vi "SetMotors.vi"(0 "Position Motors":T4[](array[typedef]), 1 "Speed Motors":T4[](array[typedef]), 3 "Angle (radians; 0 = right)":dbl, 4 "Trigger Axes":cluster{"Left":dbl, "Right":dbl}, 5 "Strafe Joystick Axes":cluster{"X":dbl, "Y":dbl}, 6 "error in (no error)":errorcluster, 7 "Face Joystick Axes":cluster{"X":dbl, "Y":dbl}, 8 "Absolute Encoder TPR":dbl, 9 "Rotation Multipliers":T1, 10 "Rotation Angle Cluster":T2 {"FL Angle" scale=3.1416..-3.1416; "FR Angle" scale=3.1416..-3.1416; "RR Angle" scale=3.1416..-3.1416; "RL Angle" scale=3.1416..-3.1416}, 11 "Drive Train Absolute Offsets (ticks)":dbl[](array[numeric])=[-0.395, 1.11, 1.68, -1.896], 12 "Speed Multipliers":dbl=1.0) -> (13 "error out":errorcluster)   [LabVIEW 2015]
uses:
  <vilib>/Rock Robotics/WPI/MotorControl/WPI_MotorControlDeviceRef.ctl
  <vilib>/Rock Robotics/WPI/MotorControl/WPI_MotorControlType.ctl
  <vilib>/Rock Robotics/SystemInterfaces/DIO/FPGA_DIOPWMChannel.ctl
  <vilib>/Rock Robotics/WPI/PWM/WPI_PWMDeadband.ctl
  <vilib>/Rock Robotics/WPI/CAN/Jaguar/SubVIs/WPI_CANJaguar_ControlMode.ctl
  <vilib>/Rock Robotics/WPI/CAN/TalonSRX/WPI_CANTalonSRX_APIControlMode.ctl
  <vilib>/addons/control/pid/pid.llb/PID Control Input Filter (DBL).vi
  <vilib>/addons/control/pid/pid.llb/PID (DBL).vi
  <vilib>/addons/control/pid/NI_PID_pid.lvlib
panel:
  out "Position Output":dbl
  out "Speed Output":dbl
  in  "Max Wheel Speed":dbl=20000.0
  in  "Face PID Gains":T3 {"derivative time (Td, min)" format="%.3f"; "integral time (Ti, min)" format="%.3f"; "proportional gain (Kc)" format="%.3f"}
  out "Speed Chart":cluster{dbl, "Encoder Velocity":dbl}[](graph)
  out "Position Chart":cluster{dbl, "Encoder Velocity":dbl}[](graph)
  out "Speed Cluster":T11 {"RR Speed" scale=-1.0..1.0; "RL Speed" scale=-1.0..1.0; "FR Speed" scale=-1.0..1.0; "FL Speed" scale=-1.0..1.0}
  out "Angle Cluster":T2 {"FL Angle" scale=3.1416..-3.1416; "FR Angle" scale=3.1416..-3.1416; "RR Angle" scale=3.1416..-3.1416; "RL Angle" scale=3.1416..-3.1416}
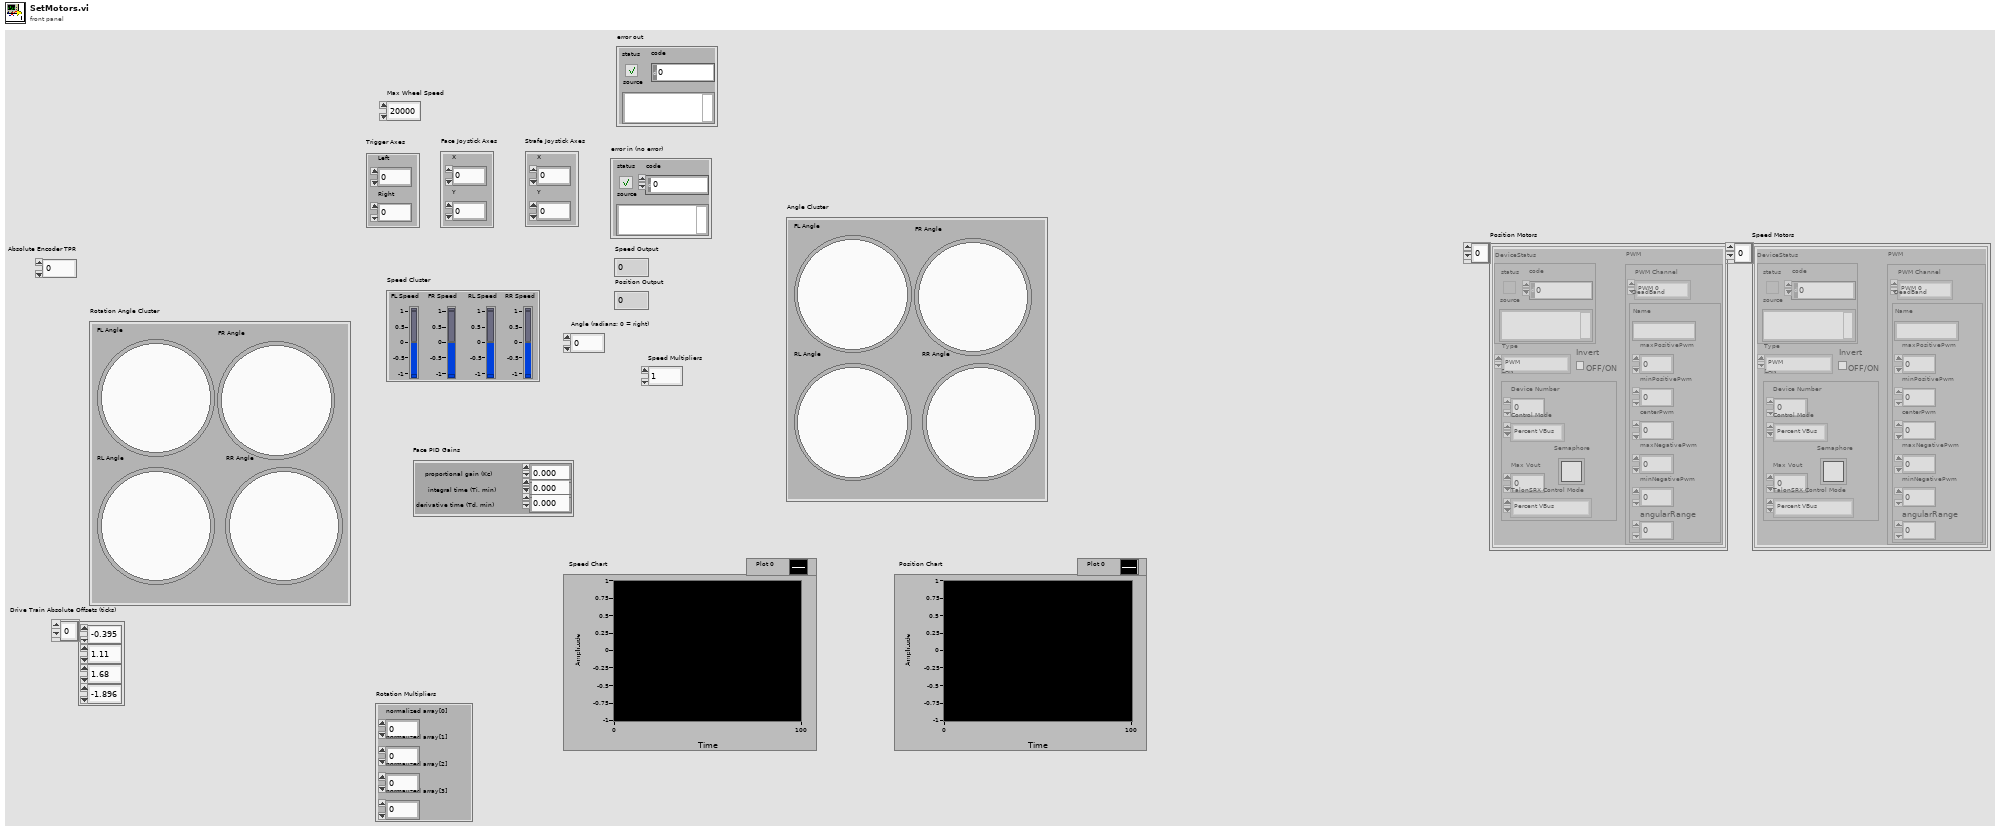
[diagram p1: front panel]
types:
  T1 = cluster{"normalized array[0]":dbl, "normalized array[1]":dbl, "normalized array[2]":dbl, "normalized array[3]":dbl}
  T2 = cluster{"FL Angle":dbl, "FR Angle":dbl, "RL Angle":dbl, "RR Angle":dbl}
  T3 = cluster{"proportional gain (Kc)":dbl, "integral time (Ti, min)":dbl, "derivative time (Td, min)":dbl}
  T4 = typedef "WPI_MotorControlDeviceRef.ctl" = cluster{"DeviceStatus":errorcluster, "Type":T5, "PWM":cluster{"PWM Channel":T6, "DeadBand":T7}, "CAN":cluster{"Device Number":u8, "Control Mode":T8, "Semaphore":T9, "Max Vout":dbl, "TalonSRX Control Mode":T10}, "Invert":bool}
  T5 = typedef "WPI_MotorControlType.ctl" = enum16{"PWM", "CAN", "CANTalonSRX"}
  T6 = typedef "FPGA_DIOPWMChannel.ctl" = enum8{"PWM 0", "PWM 1", "PWM 2", "PWM 3", "PWM 4", "PWM 5", "PWM 6", "PWM 7", "PWM 8", "PWM 9", "PWM MXP 0", "PWM MXP 1", "PWM MXP 2", "PWM MXP 3", "PWM MXP 4", "PWM MXP 5", "PWM MXP 6", "PWM MXP 7", "PWM MXP 8", "PWM MXP 9", "Invalid"}
  T7 = typedef "WPI_PWMDeadband.ctl" = cluster{"Name":string, "maxPositivePwm":i32, "minPositivePwm":i32, "centerPwm":i32, "maxNegativePwm":i32, "minNegativePwm":i32, "angularRange":u16}
  T8 = typedef "WPI_CANJaguar_ControlMode.ctl" = enum8{"Percent VBus", "Current", "Speed", "Position", "Voltage"}
  T9 = typedef "Semaphore RefNum" = refnum<k1>
  T10 = typedef "WPI_CANTalonSRX_APIControlMode.ctl" = enum8{"Percent VBus", "Speed", "Position", "Slave", "Unchanged / Invalid", "Voltage Compensation", "Current"}
  T11 = cluster{"FL Speed":dbl, "FR Speed":dbl, "RL Speed":dbl, "RR Speed":dbl}
  T12 = cluster{"[0]":dbl, "[1]":dbl, "[2]":dbl, "[3]":dbl}
  T13 = typedef "WPI_CANTalonSRX_GlobalStatus.ctl" = cluster{"Applied Throttle":dbl, "Module Enabled":bool, "CAN Error":errorcluster, "Closed Loop Error":dbl, "Forward Limit Switch Closed":bool, "Reverse Limit Switch Closed":bool, "Sensor Position":dbl, "Sensor Velocity":dbl, "Current":dbl, "Sticky Fault - Over Temp":bool, "Sticky Fault - Under Voltage":bool, "Sticky Fault - Forward Limit":bool, "Sticky Fault - Reverse Limit":bool, "Sticky Fault - Forward Soft Limit":bool, "Sticky Fault - Reverse Soft Limit":bool, "Brake is Enabled":bool, "Encoder Position":dbl, "Encoder Velocity":dbl, "Encoder Index Count":dbl, "Encoder A Pin State":bool, "Encoder B Pin State":bool, "Encoder Index Pin State":bool, "Analog In":dbl, "Analog In Velocity":dbl, "Temperature (C)":dbl, "Battery Voltage":dbl}
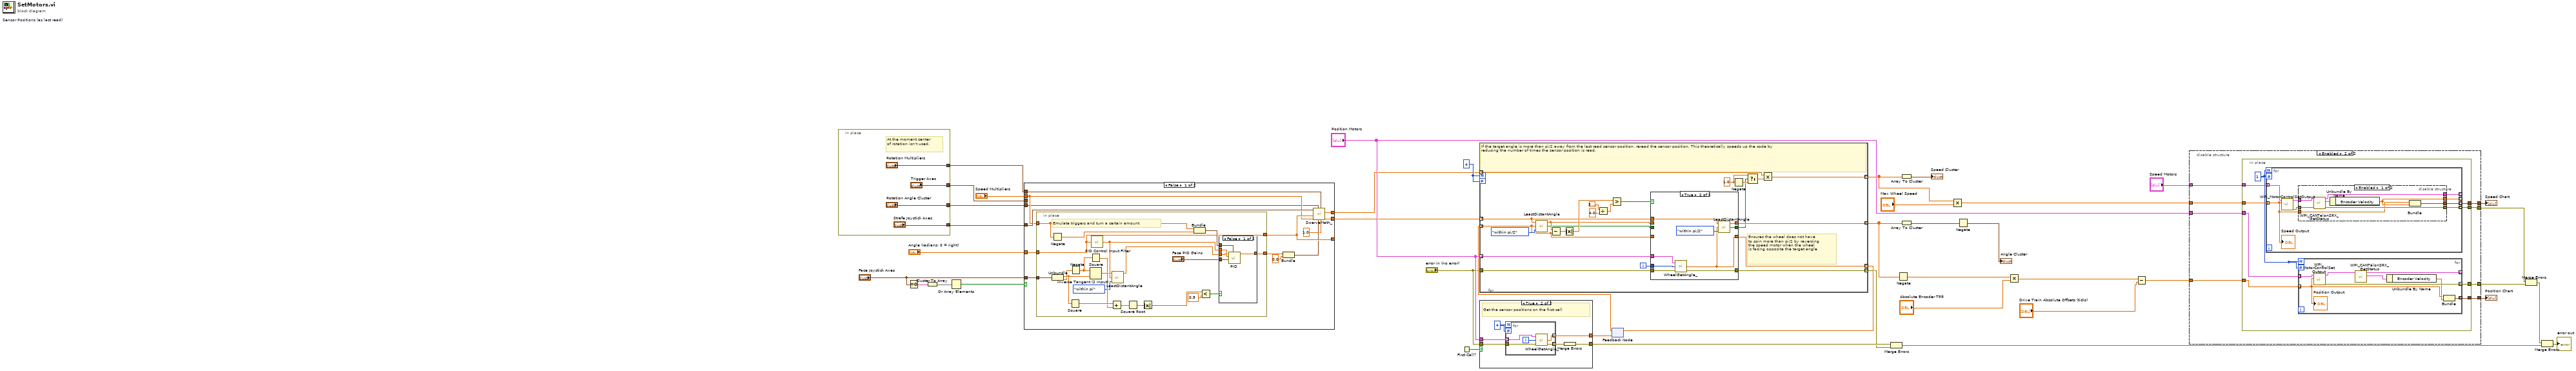
[diagram p0: block diagram]
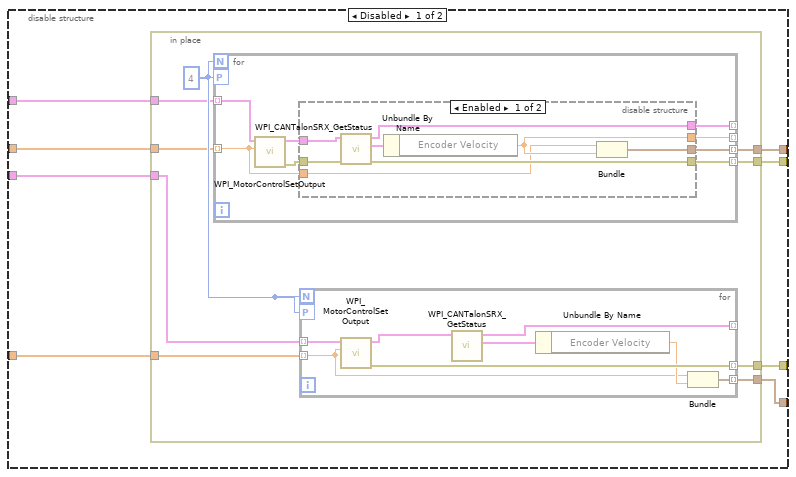
[diagram p2: hidden frame]
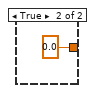
[diagram p7: hidden frame]
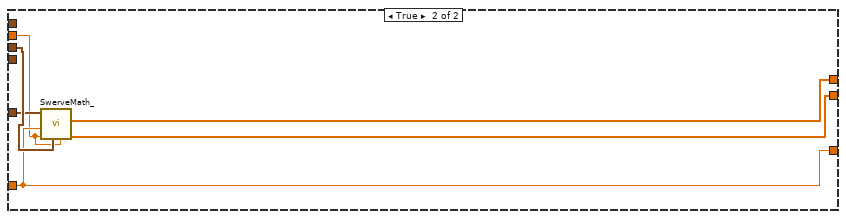
[diagram p8: hidden frame]
diagram:
  w29 = 4
  n1 = in-place {
    in-place-border: ["Strafe Joystick Axes"] -> w13
    in-place-border: ["Trigger Axes"] -> w9
    in-place-border: ["Rotation Multipliers"] -> w4
    in-place-border: ["Rotation Angle Cluster"] -> w3
    # "At the moment center\nof rotation isn't used."
  }
  n2 = Equal To 0?(x="Face Joystick Axes") -> (x = 0?=w32:cluster{"X":bool, "Y":bool})
  n3 = Cluster To Array(cluster=w32) -> (array=w30:bool[])
  n4 = Or Array Elements(Boolean array=w30) -> (logical OR=w31:bool)
  n5 = case shown="False" w31 {
    tunnel: "Face Joystick Axes" -> [w58 _]
    tunnel: [w53 w89] -> _
    tunnel: "Angle (radians; 0 = right)" -> [w57 w89]
    tunnel: w13 -> [w54 w90]
    tunnel: [w51 w88] -> w11
    tunnel: [w50 w87] -> w12
    tunnel: "Speed Multipliers" -> [w48 w86]
    tunnel: w9 -> [_ w91]
    tunnel: w4 -> [w47 _]
    tunnel: w3 -> [w46 _]
    frame False {
      n6 = in-place {
        in-place-border: [w79] -> w56
        in-place-border: [w60] -> w53
        in-place-border: w58 -> [w62]
        in-place-border: w57 -> [w60]
        in-place-border: w48 -> [w59]
        # "Emulate triggers and turn a certain amount"
        n7 = Negate(x=w59) -> (-x=w68:dbl)
        n8 = Unbundle(w62) -> ("X"=w73:dbl, "Y"=w72:dbl)
        n9 = Square(x=w73) -> (x^2=w77:dbl)
        n10 = Negate(x=w72) -> (-x=w69:dbl)
        n11 = Square(x=w69) -> (x^2=w76:dbl)
        n12 = Inverse Tangent (2 Input)(1:w73, 2:w69) -> (0:w65:dbl)
        n13 = call-poly <vilib>:"PID Control Input Filter.vi"("input"=w60) -> ("output"=w63:dbl)  [unwired: 4 in]
        n14 = Add(x=w77, y=w76) -> (x+y=w75:dbl)
        n15 = call "LeastDistantAngle.vi"("Enum"=enum16{"within pi", "within pi/2"}."within pi", "Current angle"=w63, "target angle (between pi and -pi)"=w65) -> ("output angle"=w61:dbl)  [unwired: 2 out]
        n16 = Square Root(x=w75) -> (sqrt(x)=w74:dbl)
        n17 = Absolute Value(x=w74) -> (abs(x)=w70:dbl)
        n18 = Bundle("Speed Multipliers"=w59, w68) -> (w67:cluster{"Speed Multipliers":dbl, dbl})  [unwired: 1 in]
        n19 = Less?(x=w70, y=0.5) -> (x < y?=w64:bool)
        n20 = case shown="False" w64 {
          tunnel: [w84 0.0 ("output")] -> w79
          tunnel: "Face PID Gains" -> [w83 _]
          tunnel: w67 -> [w82 _]
          tunnel: w63 -> [w81 _]
          tunnel: w61 -> [w80 _]
          frame False {
            n21 = call-poly <vilib>:"PID.vi"("output range"=w82, "PID gains"=w83, "process variable"=w81, "setpoint"=w80) -> ("output"=w84:dbl)  [unwired: 6 in, 1 out]
          }
          frame True {
          }
        }
      }
      n22 = Bundle("output"=w56, 0.0) -> (w52:cluster{"output":dbl, dbl})  [unwired: 1 in]
      n23 = call "SwerveMath_.vi"("Rotation Multiplier"=1.0, "Rotation Multipliers"=w47, "Trigger Axes/Turn Speed"=w52, "Rotation Angle Cluster"=w46, "Strafe Multiplier"=w48, "Angle (radians; 0 = right)"=w53, "Strafe Joystick Axes"=w54) -> ("Motor Angles"=w50:dbl[], "Motor Speeds"=w51:dbl[])  [unwired: 3 in]
    }
    frame True {
      n24 = call "SwerveMath_.vi"("Rotation Multiplier"=w86, "Trigger Axes/Turn Speed"=w91, "Strafe Multiplier"=w86, "Angle (radians; 0 = right)"=w89, "Strafe Joystick Axes"=w90) -> ("Motor Angles"=w87:dbl[], "Motor Speeds"=w88:dbl[])  [unwired: 5 in]
    }
  }
  n25 = First Call?() -> (First Call?: T/F=w26:bool)
  n26 = case shown="True" w26 {
    tunnel: "error in (no error)" -> [w92 w98]
    tunnel: [w92 w97] -> w25
    tunnel: "Position Motors" -> [_ w96]
    tunnel: [_ w95] -> w22
    frame False {
    }
    frame True {
      w93 = 4
      # "Get the sensor positions on the first call"
      n27 = for {
        N: w93 -> [_]
        tunnel: [w102] -> w95 mode=indexing
        tunnel: w98 -> [w103]
        tunnel: [w101] -> w94 mode=indexing
        workers-P: w93 -> [_]
        tunnel: w96 -> [w100] mode=indexing
        i -> [w99]
        n28 = call "WheelGetAngle_.vi"("error in (no error)"=w103, "Wheel"=w99, "CAN Talon SRX Ref"=w100) -> ("error out"=w101:errorcluster, "Sensor Position (rad)"=w102:dbl)  [unwired: 1 out]
      }
      n29 = Merge Errors(w94) -> (w97:errorcluster)
    }
  }
  n30 = feedback #1 "Sensor Positions (as last read)"(w22) -> (w27:dbl[])
  n31 = for {
    N: w29 -> [_]
    workers-P: w29 -> [_]
    tunnel: [w126] -> w28 mode=indexing
    tunnel: w12 -> [w104] mode=indexing
    tunnel: w27 -> [w115] mode=indexing
    tunnel: "error in (no error)" -> [w125]
    tunnel: [w124] -> w23 mode=indexing
    tunnel: "Position Motors" -> [w122] mode=indexing
    tunnel: w11 -> [w110] mode=indexing
    tunnel: [w109] -> w20 mode=indexing
    tunnel: [w107] -> w16 mode=indexing
    i -> [w121]
    w113 = 1.0 ("t")
    # "Ensures the wheel does not have\nto spin more than pi/2 by reversing\nthe speed motor when the wheel\nis facing opposite the target angle"
    # "If the target angle is more than pi/2 away from the last read sensor position, reread the sensor position. This theoretically speeds up the code by\nreducing the number of times the sensor position is read."
    n32 = call "LeastDistantAngle.vi"("Enum"=enum16{"within pi", "within pi/2"}."within pi/2", "Current angle"=w115, "target angle (between pi and -pi)"=w104) -> ("Reverse?"=w105:bool, "output angle"=w108:dbl)  [unwired: 1 out]
    n33 = Subtract(x=w108, y=w115) -> (x-y=w114:dbl)
    n34 = Absolute Value(x=w114) -> (abs(x)=w120:dbl)
    n35 = Divide(x=3.141592653589793, y=4.0) -> (x/y=w117:dbl)
    n36 = Greater?(x=w120, y=w117) -> (0:w123:bool)
    n37 = case shown="True" w123 {
      tunnel: [w130 w131] -> w126
      tunnel: w115 -> [w130 _]
      tunnel: w125 -> [w129 w133]
      tunnel: [w129 w132] -> w124
      tunnel: w122 -> [_ w135]
      tunnel: w121 -> [_ w134]
      tunnel: w108 -> [w128 _]
      tunnel: [w128 w136] -> w107
      tunnel: [w127 w137] -> w106
      tunnel: w105 -> [w127 _]
      tunnel: w104 -> [_ w138]
      frame False {
      }
      frame True {
        n38 = call "WheelGetAngle_.vi"("error in (no error)"=w133, "Wheel"=w134, "CAN Talon SRX Ref"=w135) -> ("error out"=w132:errorcluster, "Sensor Position (rad)"=w131:dbl)  [unwired: 1 out]
        n39 = call "LeastDistantAngle.vi"("Enum"=enum16{"within pi", "within pi/2"}."within pi/2", "Current angle"=w131, "target angle (between pi and -pi)"=w138) -> ("Reverse?"=w137:bool, "output angle"=w136:dbl)  [unwired: 1 out]
      }
    }
    n40 = Negate(x=w113) -> (-x=w112:dbl)
    n41 = Select(t=w113, s=w106, f=w112) -> (s? t:f=w111:dbl)
    n42 = Multiply(x=w110, y=w111) -> (x*y=w109:dbl)
  }
  n43 = feedback-in #1(w28) -> ()
  n44 = Merge Errors(w25, w23) -> (w7:errorcluster)
  n45 = Negate(x=w16) -> (-x=w15:dbl[])
  n46 = Array To Cluster(array=w20) -> (cluster=→"Speed Cluster":T12)
  n47 = Array To Cluster(array=w16) -> (cluster=w17:T12)
  n48 = Multiply(x=w20, y="Max Wheel Speed") -> (x*y=w36:dbl[])
  n49 = Negate(x=w17) -> (-x=→"Angle Cluster":T12)
  n50 = Multiply(x=w15, y="Absolute Encoder TPR") -> (x*y=w19:dbl[])
  n51 = Subtract(x=w19, y="Drive Train Absolute Offsets (ticks)") -> (x-y=w37:dbl[])
  n52 = disable-structure shown="Enabled" {
    disable-tunnel: [w147 w189] -> w41
    disable-tunnel: [w146 w188] -> w40
    disable-tunnel: [w145 w187] -> w39
    disable-tunnel: [w144 w186] -> w38
    disable-tunnel: w37 -> [w143 w185]
    disable-tunnel: w36 -> [w142 w184]
    disable-tunnel: "Position Motors" -> [w141 w183]
    disable-tunnel: "Speed Motors" -> [w140 w182]
    frame Disabled {
      n53 = in-place {
        in-place-border: [w156] -> w147
        in-place-border: [w154] -> w146
        in-place-border: [w153] -> w145
        in-place-border: [w152] -> w144
        in-place-border: w143 -> [w151]
        in-place-border: w142 -> [w150]
        in-place-border: w141 -> [w149]
        in-place-border: w140 -> [w148]
        w155 = 4
        n54 = for {
          N: w155 -> [_]
          tunnel: [w170] -> w156 mode=indexing
          workers-P: w155 -> [_]
          tunnel: w148 -> [w172] mode=indexing
          tunnel: [w168] -> _ mode=indexing
          tunnel: [w167] -> w153 mode=indexing
          tunnel: w150 -> [w166] mode=indexing
          tunnel: [w165] -> _ mode=indexing
          n55 = call <vilib>:"WPI_MotorControlSetOutput.vi"("Output"=w166, "MotorControlDevRef"=w172) -> ("error out"=w171:errorcluster, "MotorControlDevRef"=w169:T4)  [unwired: 7 in, 1 out]
          n56 = disable-structure shown="Enabled" {
            disable-tunnel: w171 -> [w180 w181]
            disable-tunnel: [w179 w181] -> w170
            disable-tunnel: w169 -> [w178 _]
            disable-tunnel: [w176 _] -> w168
            disable-tunnel: [w174 _] -> w167
            disable-tunnel: w166 -> [w175 _]
            disable-tunnel: [w173 _] -> w165
            frame Enabled {
              n57 = call <vilib>:"WPI_CANTalonSRX_GetStatus.vi"("error in (no error)"=w180, "CAN Talon SRX Ref"=w178) -> ("error out"=w179:errorcluster, "Talon SRX Status"=w177:T13, "CAN Talon SRX Ref Out"=w173:T4)  [unwired: 7 in]
              n58 = Unbundle By Name(w177) -> ("Encoder Velocity"=w176:dbl)
              n59 = Bundle(w175, "Encoder Velocity"=w176) -> (w174:cluster{dbl, "Encoder Velocity":dbl})  [unwired: 1 in]
            }
            frame Disabled {
            }
          }
        }
        n60 = for {
          N: w155 -> [_]
          workers-P: w155 -> [_]
          tunnel: w149 -> [w164] mode=indexing
          tunnel: w151 -> [w159] mode=indexing
          tunnel: [w163] -> w154 mode=indexing
          tunnel: [w158] -> w152 mode=indexing
          tunnel: [w157] -> _ mode=indexing
          n61 = call <vilib>:"WPI_MotorControlSetOutput.vi"("Output"=w159, "MotorControlDevRef"=w164) -> ("error out"=w163:errorcluster, "MotorControlDevRef"=w161:T4)  [unwired: 7 in, 1 out]
          n62 = call <vilib>:"WPI_CANTalonSRX_GetStatus.vi"("CAN Talon SRX Ref"=w161) -> ("Talon SRX Status"=w162:T13, "CAN Talon SRX Ref Out"=w157:T4)  [unwired: 8 in, 1 out]
          n63 = Unbundle By Name(w162) -> ("Encoder Velocity"=w160:dbl)
          n64 = Bundle(w159, "Encoder Velocity"=w160) -> (w158:cluster{dbl, "Encoder Velocity":dbl})  [unwired: 1 in]
        }
      }
    }
    frame Enabled {
      n65 = in-place {
        in-place-border: [w198] -> w189
        in-place-border: [w196] -> w188
        in-place-border: [w195] -> w187
        in-place-border: [w194] -> w186
        in-place-border: w185 -> [w193]
        in-place-border: w184 -> [w192]
        in-place-border: w183 -> [w191]
        in-place-border: w182 -> [w190]
        w197 = 1
        n66 = for {
          N: w197 -> [_]
          tunnel: [w212] -> w198 mode=indexing
          workers-P: w197 -> [_]
          tunnel: w190 -> [w214] mode=indexing
          tunnel: [w210] -> _ mode=indexing
          tunnel: [w209] -> w195 mode=indexing
          tunnel: w192 -> [w208] mode=indexing
          tunnel: [w207] -> _ mode=indexing
          n67 = call <vilib>:"WPI_MotorControlSetOutput.vi"("Output"=w208, "MotorControlDevRef"=w214) -> ("error out"=w213:errorcluster, "MotorControlDevRef"=w211:T4)  [unwired: 7 in, 1 out]
          n68 = disable-structure shown="Enabled" {
            disable-tunnel: w213 -> [w222 w223]
            disable-tunnel: [w221 w223] -> w212
            disable-tunnel: w211 -> [w220 _]
            disable-tunnel: [w218 _] -> w210
            disable-tunnel: [w216 _] -> w209
            disable-tunnel: w208 -> [w217 _]
            disable-tunnel: [w215 _] -> w207
            frame Enabled {
              n69 = call <vilib>:"WPI_CANTalonSRX_GetStatus.vi"("error in (no error)"=w222, "CAN Talon SRX Ref"=w220) -> ("error out"=w221:errorcluster, "Talon SRX Status"=w219:T13, "CAN Talon SRX Ref Out"=w215:T4)  [unwired: 7 in]
              n70 = Unbundle By Name(w219) -> ("Encoder Velocity"=w218:dbl)
              n71 = Bundle(w217, "Encoder Velocity"=w218) -> (w216:cluster{dbl, "Encoder Velocity":dbl})  [unwired: 1 in]
            }
            frame Disabled {
            }
          }
          "Speed Output" <- w208
        }
        n72 = for {
          N: w197 -> [_]
          workers-P: w197 -> [_]
          tunnel: w191 -> [w206] mode=indexing
          tunnel: w193 -> [w199] mode=indexing
          tunnel: [w205] -> w196 mode=indexing
          tunnel: [w201] -> w194 mode=indexing
          tunnel: [w200] -> _ mode=indexing
          n73 = call <vilib>:"WPI_MotorControlSetOutput.vi"("Output"=w199, "MotorControlDevRef"=w206) -> ("error out"=w205:errorcluster, "MotorControlDevRef"=w203:T4)  [unwired: 7 in, 1 out]
          n74 = call <vilib>:"WPI_CANTalonSRX_GetStatus.vi"("CAN Talon SRX Ref"=w203) -> ("Talon SRX Status"=w204:T13, "CAN Talon SRX Ref Out"=w200:T4)  [unwired: 8 in, 1 out]
          n75 = Unbundle By Name(w204) -> ("Encoder Velocity"=w202:dbl)
          n76 = Bundle(w199, "Encoder Velocity"=w202) -> (w201:cluster{dbl, "Encoder Velocity":dbl})  [unwired: 1 in]
          "Position Output" <- w199
        }
      }
    }
  }
  "Speed Chart" <- w39
  "Position Chart" <- w38
  n77 = Merge Errors(w41, w40) -> (w6:errorcluster)
  n78 = Merge Errors(w6, w7) -> (→"error out":errorcluster)
